vi "rad_Retrieve RAD AppImage Properties from Target.vi"(5 "password":string, 7 "user (admin)":string="admin", 8 "error in (no error)":errorcluster, 10 "App Images Temp Folder":path=path "C:/dev/Architectures/Reference Designs/Application Deployment and Replication/Application Deployment Utility/trunk/source/Application Images/_temp", 11 "Target settings":T1={"Hostname"="", "Serial number"="", "Product name"="", "Product code"=0, "System status"="", "Credential type"=enum."None/Unlocked", "User added?"=FALSE, "Primary NIC"={"MAC address"="", "IP Address Request Mode"=2, "IP address"="", "Subnet mask"="", "Gateway"="", "DNS server"=""}} {"Primary NIC"."IP Address Request Mode" items=["Static"=1, "DHCP/Link-Local"=2, "Link-Local Only"=4, "DHCP Only"=8]}) -> (0 "error out":errorcluster, 3 "RAD AppImage Properties":T3)   [LabVIEW 2014]
uses:
  TypeDefs/rad_Application Image Properties.ctl
  TypeDefs/rad_FPGA Properties.ctl
  TypeDefs/rad_FPGA Flash Properties.ctl
  Targets/TypeDefs/rad_Target Information.ctl
  Targets/TypeDefs/rad_Target Network Settings.ctl
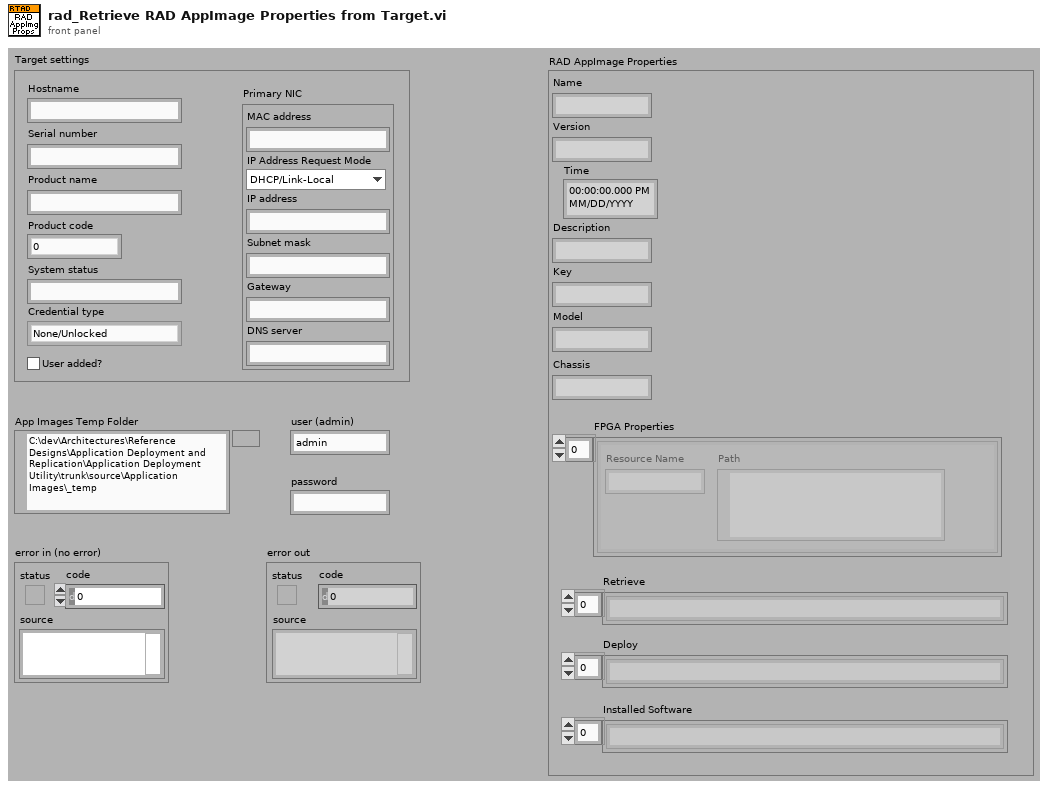
[diagram p1: front panel]
types:
  T1 = typedef "rad_Target Information.ctl" = cluster{"Hostname":string, "Serial number":string, "Product name":string, "Product code":i32, "System status":string, "Credential type":enum16{"None/Unlocked", "FTP Password", "NIAuth Credentials"}, "User added?":bool, "Primary NIC":T2}
  T2 = typedef "rad_Target Network Settings.ctl" = cluster{"MAC address":string, "IP Address Request Mode":i32, "IP address":string, "Subnet mask":string, "Gateway":string, "DNS server":string}
  T3 = typedef "rad_Application Image Properties.ctl" = cluster{"Name":string, "Version":string, "Time":timestamp, "Description":string, "Key":string, "Chassis":string, "FPGA Properties":T4, "Model":string, "Retrieve":string[], "Deploy":string[], "Installed Software":string[]}
  T4 = typedef "rad_FPGA Properties.ctl" = T5[]
  T5 = typedef "rad_FPGA Flash Properties.ctl" = cluster{"Resource Name":string, "Path":path}
  T6 = enum16{"None/Unlocked", "FTP Password", "NIAuth Credentials"}
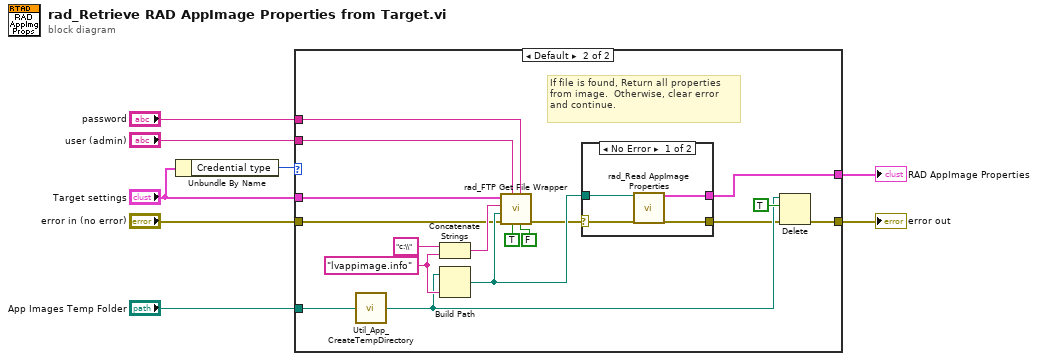
[diagram p0: block diagram]
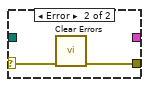
[diagram p3: hidden frame]
diagram:
  n1 = Unbundle By Name("Target settings") -> ("Credential type"=w1:T6)
  n2 = case shown="Default" w1 {
    tunnel: "user (admin)" -> [_ w23]
    tunnel: "password" -> [_ w22]
    tunnel: "App Images Temp Folder" -> [_ w14]
    tunnel: "error in (no error)" -> [w9 w13]
    tunnel: [w9 w12] -> w4
    tunnel: [_ w11] -> w3
    tunnel: "Target settings" -> [_ w10]
    frame "NIAuth Credentials" {
      # "On a pure NIAuth target, we get the settings\ndirectly from NI System Configuration API."
    }
    frame Default {
      w24 = "lvappimage.info" ("string")
      # "If file is found, Return all properties from image.  Otherwise, clear error\nand continue."
      n3 = call "Util_App_CreateTempDirectory.vi"("TempFolderPath"=w14) -> ("TempFolderPath_out"=w17:path)
      n4 = Concatenate Strings("c:\\" ("remote path"), w24) -> (w25:string)
      n5 = Build Path(base path=w17, name or relative path=w24) -> (appended path=w21:path)
      n6 = call "rad_FTP Get File Wrapper.vi"("active (F)"=FALSE ("active (T)"), "password"=w22, "binary (T)"=TRUE ("binary (F)"), "user (admin)"=w23, "error in (no error)"=w13, "local path"=w21, "remote path"=w25, "Target settings"=w10) -> ("error out"=w15:errorcluster)  [unwired: 3 in]
      n7 = case shown="No Error" w15 {
        selector: w15 -> [w27 w31]
        tunnel: w21 -> [w30 _]
        tunnel: [w28 w32] -> w16
        tunnel: [w29 _] -> w11
        frame No Error {
          n8 = call "rad_Read AppImage Properties.vi"("AppImage Properties Path"=w30, "error in (no error)"=w27) -> ("AppImage Properties"=w29:T3, "error out"=w28:errorcluster)  [unwired: 12 in, 4 out]
        }
        frame Error {
          n9 = call <vilib>:"Clear Errors.vi"("error in (no error)"=w31) -> ("error out"=w32:errorcluster)  [unwired: 5 in, 1 out]
        }
      }
      n10 = Delete(path (use dialog)=w17, entire hierarchy (F)=TRUE, error in=w16) -> (error out=w12:errorcluster)  [unwired: 2 in, 2 out]
    }
  }
  "error out" <- w4
  "RAD AppImage Properties" <- w3
